vi "or(Web).vi"(7 "LabVIEW Web Service Request":refnum<class "Web Request.lvclass">, 9 "z":bool, 10 "y":bool, 11 "x":bool) -> (2 "number":u32, 3 "x.or.y.or.z":string)   [LabVIEW 2017]
uses:
  <vilib>/wsapi/Web Request.lvclass
panel:
  # "Use the Web Service Request input terminal to call the VIs on the Web Services palette. Do not remove it from the connector pane unless you don't need access to the palette."
  # "Each additional control wired to the connector pane will be available as an input in the URL. To include an indicator in terminal-mode output (the default setting), it must also be wired to the connector pane."
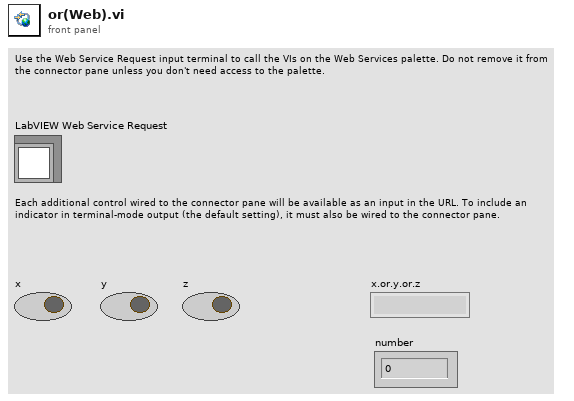
[diagram p1: front panel]
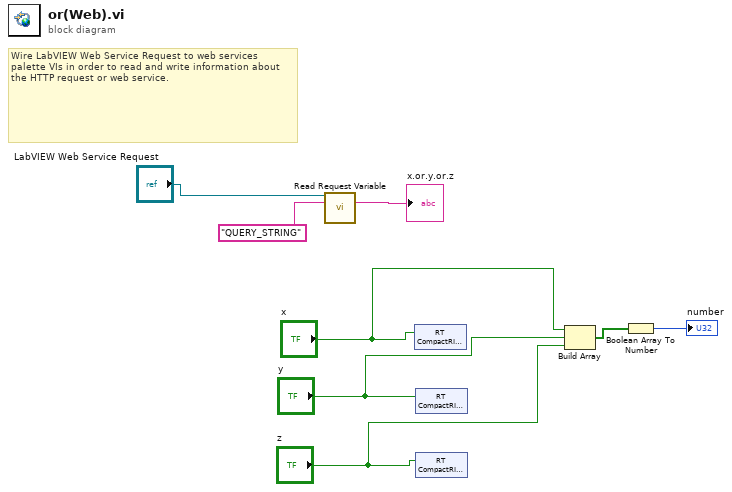
[diagram p0: block diagram]
diagram:
  # "Wire LabVIEW Web Service Request to web services palette VIs in order to read and write information about the HTTP request or web service."
  n1 = call <vilib>:"Read Request Variable.vi"("LabVIEW Web Service Request"="LabVIEW Web Service Request", "variable name"="QUERY_STRING") -> ("value"=→"x.or.y.or.z":string)  [unwired: 11 in, 2 out]
  n2 = shared-variable "RT CompactRIO Target \\variable.lvlib\\X"("x") -> ()  [unwired: 1 in, 1 out]
  n3 = shared-variable "RT CompactRIO Target \\variable.lvlib\\Y"("y") -> ()  [unwired: 1 in, 1 out]
  n4 = shared-variable "RT CompactRIO Target \\variable.lvlib\\Z"("z") -> ()  [unwired: 1 in, 1 out]
  n5 = Build Array("x", "y", "z") -> (w2:bool[])
  n6 = Boolean Array To Number(Boolean array=w2) -> (number=→"number":u32)
